vi "CLD 12 Sequencer State Machine solution.vi"() -> ()   [LabVIEW 2018]
doc: "CLD 12: Sequences boolean values in the order they are loaded from the file."
uses:
  CLD 12 Sequencer Enum.ctl
  CLD 12 Data Cluster.ctl
  CLD12 Timer Enum.ctl
panel:
  out "Current Time Target":dbl
  in  "error in (no error)":errorcluster
  out "error out":errorcluster
  in  "Stop Button":bool
  out "Time Elapsed":dbl
  out "Switch 3":bool
  out "Switch 2":bool
  out "Switch 1":bool
  in  "Start":bool
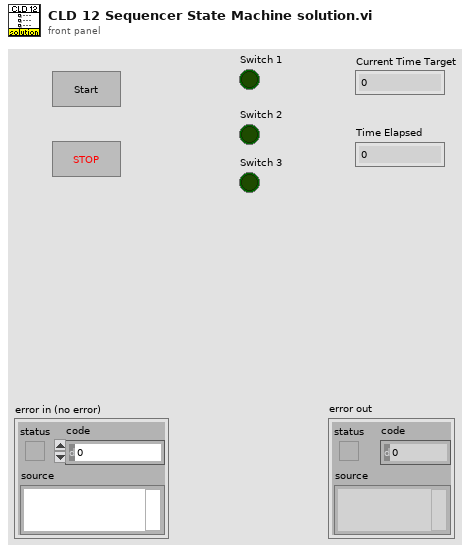
[diagram p1: front panel]
types:
  T1 = typedef "CLD 12 Data Cluster.ctl" = cluster{"Command":T2, "Time Value":dbl, "Boolean 1":bool, "Boolean 2":bool, "Boolean 3":bool}
  T2 = typedef "CLD 12 Sequencer Enum.ctl" = enum16{"Initialize", "SetTime", "RunState1", "Runstate2", "Idle", "Start"}
  T3 = typedef "CLD12 Timer Enum.ctl" = enum16{"Start Timer", "Read Time", "Pause", "UnPause", "Reset Timer"}
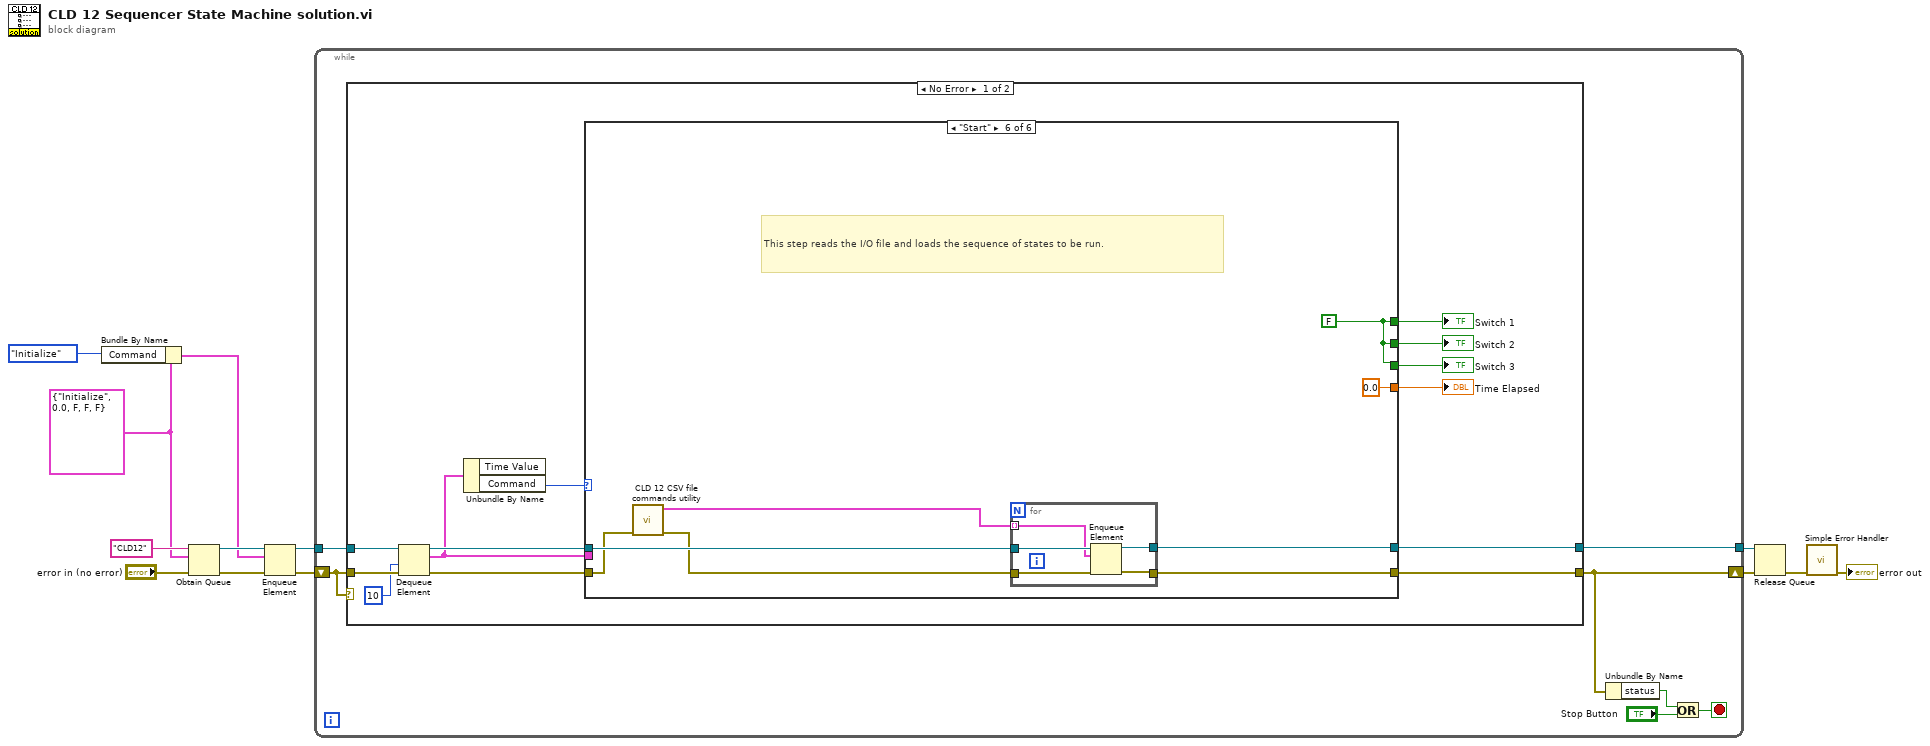
[diagram p0: block diagram]
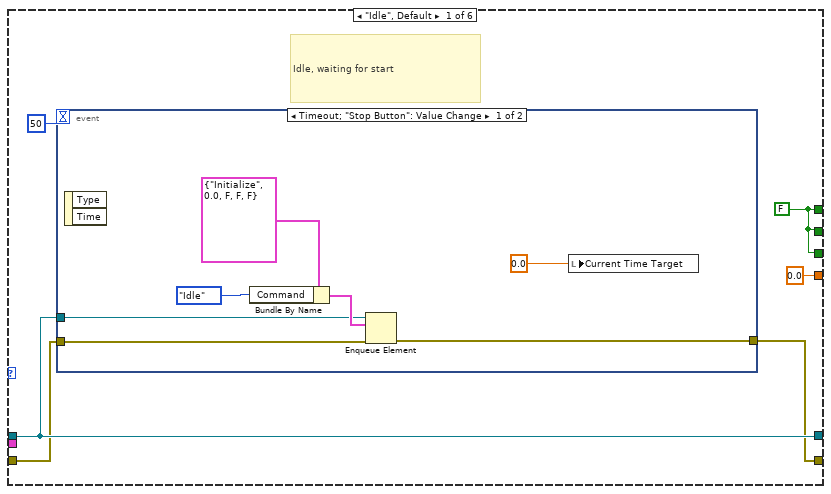
[diagram p2: hidden frame]
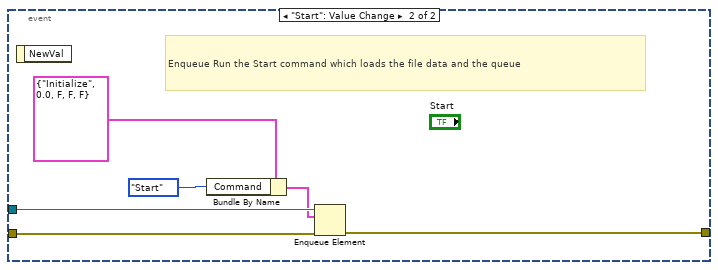
[diagram p3: hidden frame]
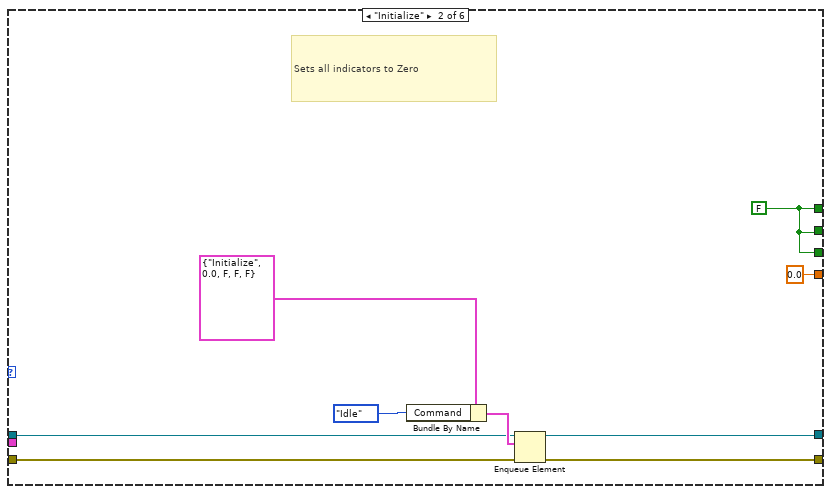
[diagram p4: hidden frame]
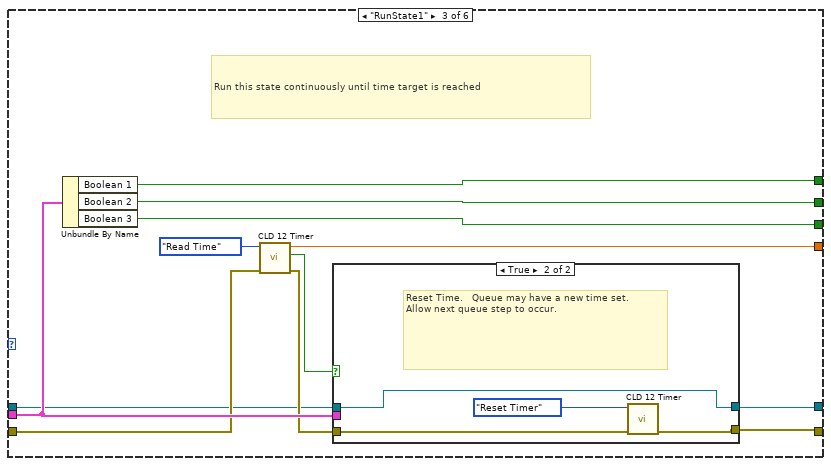
[diagram p5: hidden frame]
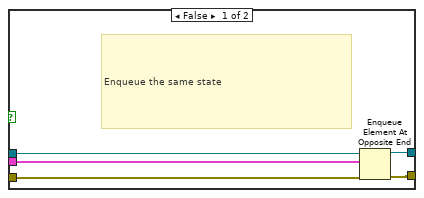
[diagram p6: hidden frame]
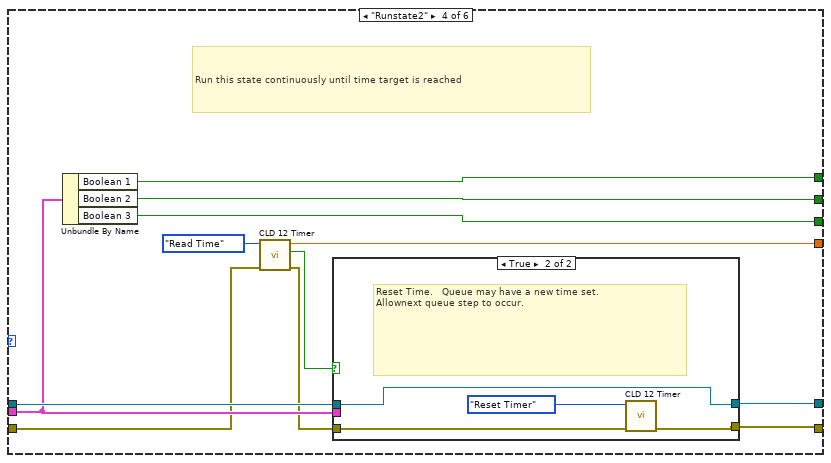
[diagram p7: hidden frame]
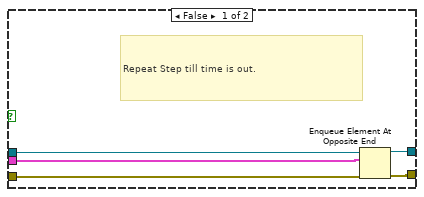
[diagram p8: hidden frame]
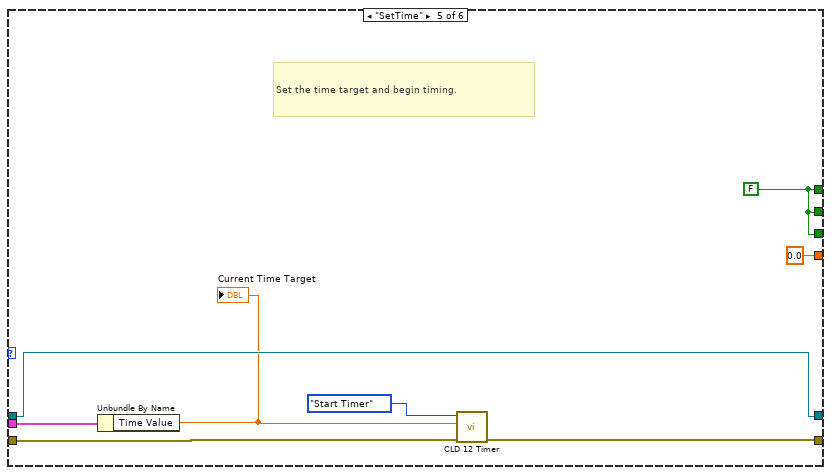
[diagram p9: hidden frame]
diagram:
  w8 = T1 {"Command"=enum."Initialize", "Time Value"=0.0, "Boolean 1"=FALSE, "Boolean 2"=FALSE, "Boolean 3"=FALSE} ("CLD 12 Data Cluster")
  n1 = Bundle By Name(cluster=w8, "Command"=CLD_12_Sequencer_Enum."Initialize" ("CLD 12 Sequencer Control")) -> (w7:T1)
  n2 = Obtain Queue(name (unnamed)="CLD12", element data type=w8, error in (no error)="error in (no error)") -> (queue out=w11:refnum<queue>, error out=w13:errorcluster)  [unwired: 2 in, 1 out]
  n3 = Enqueue Element(queue=w11, element=w7, error in (no error)=w13) -> (queue out=w10:refnum<queue>, error out=w12:errorcluster)  [unwired: 1 in, 1 out]
  n4 = while {
    tunnel: w10 -> [w20]
    shift-right: [w16] -> w5
    shift-left: w12 -> [w18]
    tunnel: [w15] -> w4
    stop <- w17 stop-if-true
    n5 = case shown="No Error" w18 {
      tunnel: [w33 w126] -> w16
      tunnel: w20 -> [w32 w125]
      tunnel: w18 -> [w30 w126]
      tunnel: [w22 w125] -> w15
      frame No Error {
        n6 = Dequeue Element(queue=w32, timeout in ms (-1)=10, error in (no error)=w30) -> (queue out=w31:refnum<queue>, element=w27:T1, error out=w29:errorcluster)  [unwired: 1 out]
        n7 = Unbundle By Name(w27) -> ("Command"=w28:T2)  [unwired: 1 out]
        n8 = case shown="\"Start\"" w28 {
          tunnel: [w36 w57 w67 w87 w110 w118] -> w33
          tunnel: w29 -> [w37 w58 w66 w86 w111 w116]
          tunnel: w31 -> [w39 w54 w64 w94 w106 w119]
          tunnel: w27 -> [_ _ w68 w88 w109 _]
          tunnel: [w35 w56 w73 w93 w108 w114] -> w26
          tunnel: [w35 w56 w72 w92 w108 w114] -> w25
          tunnel: [w35 w56 w71 w91 w108 w114] -> w24
          tunnel: [0.0 ("Elapsed Time (s.ss)") 0.0 ("Elapsed Time (s.ss)") w70 w90 0.0 ("Elapsed Time (s.ss)") 0.0 ("Elapsed Time (s.ss)")] -> w23
          tunnel: [w39 w53 w63 w84 w106 w112] -> w22
          frame "Idle", Default {
            w35 = FALSE ("Boolean 1")
            # "Idle, waiting for start"
            n9 = event shown="[0] Timeout;  \"Stop Button\": Value Change" {
              selector: _ -> [_ _]
              dyn-events: _ -> [_ _]
              timeout: 50 -> [_ _]
              tunnel: w37 -> [w42 w52]
              tunnel: w39 -> [w43 w51]
              tunnel: [w41 w47] -> w36
              event Timeout; "Stop Button": Value Change {
                n10 = event-data() -> ()  [unwired: 1 in, 2 out]
                n11 = Bundle By Name(cluster=T1 {"Command"=enum."Initialize", "Time Value"=0.0, "Boolean 1"=FALSE, "Boolean 2"=FALSE, "Boolean 3"=FALSE} ("CLD 12 Data Cluster"), "Command"=CLD_12_Sequencer_Enum."Idle" ("CLD 12 Sequencer Control")) -> (w44:T1)
                n12 = Enqueue Element(queue=w43, element=w44, error in (no error)=w42) -> (error out=w41:errorcluster)  [unwired: 1 in, 2 out]
                n13 = local write "Current Time Target"(0.0 ("Current Time Value")) -> ()
              }
              event "Start": Value Change {
                # "Enqueue Run the Start command which loads the file data and the queue"
                n14 = event-data() -> ()  [unwired: 1 in, 1 out]
                n15 = Bundle By Name(cluster=T1 {"Command"=enum."Initialize", "Time Value"=0.0, "Boolean 1"=FALSE, "Boolean 2"=FALSE, "Boolean 3"=FALSE} ("CLD 12 Data Cluster"), "Command"=CLD_12_Sequencer_Enum."Start" ("CLD 12 Sequencer Control")) -> (w48:T1)
                n16 = Enqueue Element(queue=w51, element=w48, error in (no error)=w52) -> (error out=w47:errorcluster)  [unwired: 1 in, 2 out]
              }
            }
          }
          frame "Initialize" {
            w56 = FALSE ("Boolean 1")
            # "Sets all indicators to Zero"
            n17 = Bundle By Name(cluster=T1 {"Command"=enum."Initialize", "Time Value"=0.0, "Boolean 1"=FALSE, "Boolean 2"=FALSE, "Boolean 3"=FALSE} ("CLD 12 Data Cluster"), "Command"=CLD_12_Sequencer_Enum."Idle" ("CLD 12 Sequencer Control")) -> (w59:T1)
            n18 = Enqueue Element(queue=w54, element=w59, error in (no error)=w58) -> (queue out=w53:refnum<queue>, error out=w57:errorcluster)  [unwired: 1 in, 1 out]
          }
          frame "RunState1" {
            # "Run this state continuously until time target is reached"
            n19 = Unbundle By Name(w68) -> ("Boolean 1"=w73:bool, "Boolean 2"=w72:bool, "Boolean 3"=w71:bool)
            n20 = call "CLD 12 Timer.vi"("Error In"=w66, "CLD 12 Timer Enum"=CLD12_Timer_Enum."Read Time" ("CLD 12 Time Enum")) -> ("Error Out"=w65:errorcluster, "Has Time Elapsed ?"=w69:bool, "Elapsed Time (s.ss)"=w70:dbl)  [unwired: 7 in]
            n21 = case shown="True" w69 {
              tunnel: w64 -> [w78 w79]
              tunnel: w68 -> [w77 _]
              tunnel: w65 -> [w76 w82]
              tunnel: [w75 w81] -> w67
              tunnel: [w74 w79] -> w63
              frame False {
                # "Enqueue the same state"
                n22 = Enqueue Element At Opposite End(queue=w78, element=w77, error in (no error)=w76) -> (queue out=w74:refnum<queue>, error out=w75:errorcluster)  [unwired: 1 in, 1 out]
              }
              frame True {
                # "Reset Time.   Queue may have a new time set.\nAllow next queue step to occur."
                n23 = call "CLD 12 Timer.vi"("Error In"=w82, "CLD 12 Timer Enum"=CLD12_Timer_Enum."Reset Timer" ("CLD 12  Enum")) -> ("Error Out"=w81:errorcluster)  [unwired: 7 in, 2 out]
              }
            }
          }
          frame "Runstate2" {
            # "Run this state continuously until time target is reached"
            n24 = Unbundle By Name(w88) -> ("Boolean 1"=w93:bool, "Boolean 2"=w92:bool, "Boolean 3"=w91:bool)
            n25 = call "CLD 12 Timer.vi"("Error In"=w86, "CLD 12 Timer Enum"=CLD12_Timer_Enum."Read Time" ("CLD 12 Time Enum")) -> ("Error Out"=w85:errorcluster, "Has Time Elapsed ?"=w89:bool, "Elapsed Time (s.ss)"=w90:dbl)  [unwired: 7 in]
            n26 = case shown="True" w89 {
              tunnel: w94 -> [w99 w100]
              tunnel: w88 -> [w98 _]
              tunnel: w85 -> [w97 w103]
              tunnel: [w96 w102] -> w87
              tunnel: [w95 w100] -> w84
              frame False {
                # "Repeat Step till time is out."
                n27 = Enqueue Element At Opposite End(queue=w99, element=w98, error in (no error)=w97) -> (queue out=w95:refnum<queue>, error out=w96:errorcluster)  [unwired: 1 in, 1 out]
              }
              frame True {
                # "Reset Time.   Queue may have a new time set.\nAllownext queue step to occur."
                n28 = call "CLD 12 Timer.vi"("Error In"=w103, "CLD 12 Timer Enum"=CLD12_Timer_Enum."Reset Timer" ("CLD 12 Enum")) -> ("Error Out"=w102:errorcluster)  [unwired: 7 in, 2 out]
              }
            }
          }
          frame "SetTime" {
            w108 = FALSE ("Boolean 1")
            # "Set the time target and begin timing."
            n29 = Unbundle By Name(w109) -> ("Time Value"=w104:dbl)
            "Current Time Target" <- w104
            n30 = call "CLD 12 Timer.vi"("Error In"=w111, "Time Target (s)"=w104, "CLD 12 Timer Enum"=CLD12_Timer_Enum."Start Timer" ("CLD 12 Time Enum")) -> ("Error Out"=w110:errorcluster)  [unwired: 6 in, 2 out]
          }
          frame "Start" {
            w114 = FALSE ("Boolean 1")
            # "This step reads the I/O file and loads the sequence of states to be run."
            n31 = call "CLD 12 CSV file commands utility.vi"("Error In"=w116) -> ("Error Out"=w115:errorcluster, "Command Array Out"=w117:T1[])  [unwired: 9 in]
            n32 = for {
              tunnel: w119 -> [w124]
              tunnel: [w121] -> w118
              tunnel: w115 -> [w123]
              tunnel: w117 -> [w122] mode=indexing
              tunnel: [w120] -> w112
              n33 = Enqueue Element(queue=w124, element=w122, error in (no error)=w123) -> (queue out=w120:refnum<queue>, error out=w121:errorcluster)  [unwired: 1 in, 1 out]
            }
          }
        }
        "Time Elapsed" <- w23
        "Switch 1" <- w26
        "Switch 2" <- w25
        "Switch 3" <- w24
      }
      frame Error {
      }
    }
    n34 = Unbundle By Name(w16) -> ("status"=w14:bool)
    n35 = Or(x=w14, y="Stop Button") -> (x .or. y?=w17:bool)
  }
  n36 = Release Queue(queue=w4, error in (no error)=w5) -> (error out=w3:errorcluster)  [unwired: 1 in, 2 out]
  n37 = call <vilib>:"Simple Error Handler.vi"("error in (no error)"=w3) -> ("error out"=→"error out":errorcluster)  [unwired: 4 in, 4 out]
